vi "ex_6.vi"() -> ()   [LabVIEW 2020]
uses:
  #typedef_User.ctl
  #typedef_FGV_DatabaseAction.ctl
panel:
  out "error out":errorcluster
  in  "error in (no error)":errorcluster
  out "Users Data":T1[](array[typedef])
  in  "Database action (read data)":T2
  in  "User":T1
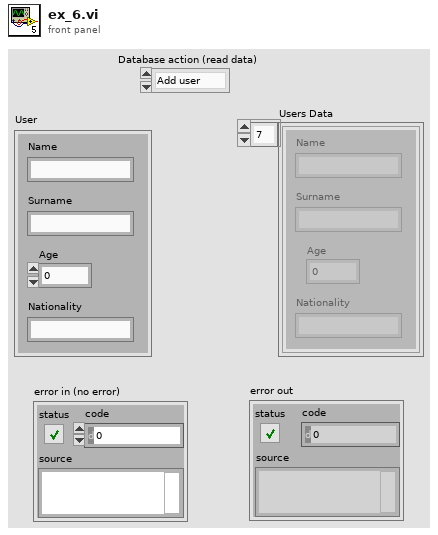
[diagram p1: front panel]
types:
  T1 = typedef "#typedef_User.ctl" = cluster{"Name":string, "Surname":string, "Age":dbl, "Nationality":string}
  T2 = typedef "#typedef_FGV_DatabaseAction.ctl" = enum16{"Add user", "Read data", "Clear data"}
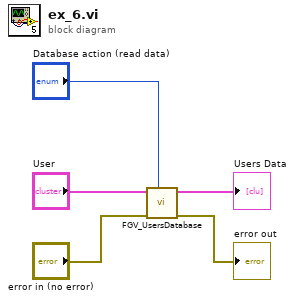
[diagram p0: block diagram]
diagram:
  n1 = call "FGV_UsersDatabase.vi"("Database action (read data)"="Database action (read data)", "error in (no error)"="error in (no error)", "User"="User") -> ("error out"=→"error out":errorcluster, "Users Data"=→"Users Data":T1[])  [unwired: 7 in]
